vi "Unregister Subsystem.vi"(8 "error in (no error)":errorcluster, 9 "RegistryKey":string, 10 "JKI SMO":refnum<class "SMO.lvclass">) -> (0 "error out":errorcluster, 2 "JKI SMO out":refnum<class "SMO.lvclass">)   [LabVIEW 2021, in "smo.lvlib" / "Registry-SMO.lvclass"]
uses:
  Registry-SMO.lvclass
  SMO/SMO.lvclass
  SMO/SMO.lvclass/SMO.ctl
  Support/Attribute.Identity/Attribute.Identity.lvclass/Attribute.Identity.ctl
  Registry-SMO.lvclass/Registry-SMO.ctl
  SMO/Private/GetVariant(Attr).vi
  Support/Attribute.Identity/Read UniqueName.vi
  Support/Attribute.Identity/Read Given Name.vi
  Support/Attribute.Identity/Read ProspectiveOwner.vi
  SMO/Private/ReftoDVR--SMO.vi
  Support/Attribute.Identity/Attribute.Identity.lvclass
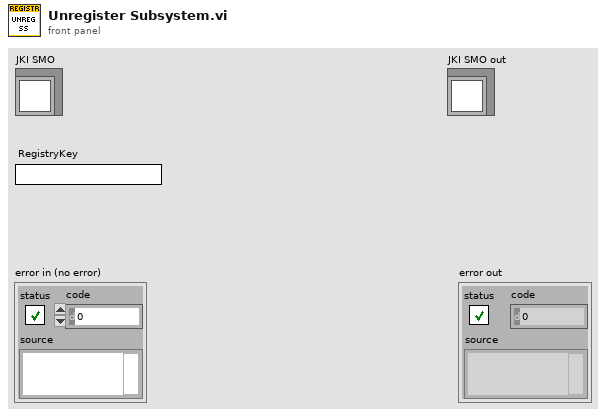
[diagram p1: front panel]
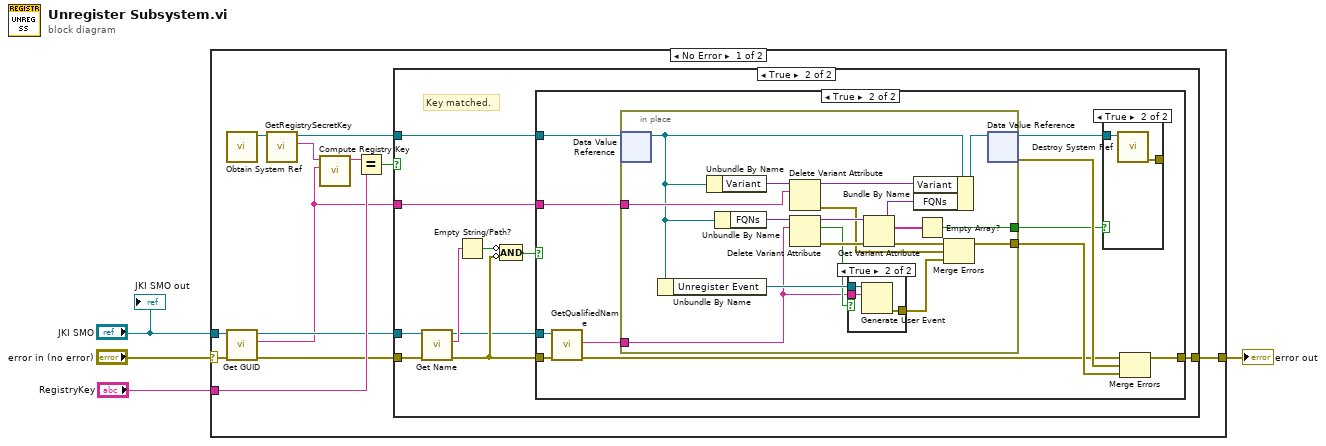
[diagram p0: block diagram]
diagram:
  n1 = case shown="No Error" "error in (no error)" {
    selector: "error in (no error)" -> [w15 w63]
    tunnel: [w16 w63] -> w3
    tunnel: "JKI SMO" -> [w14 _]
    tunnel: "RegistryKey" -> [w13 _]
    frame No Error {
      n2 = call "Obtain System Ref.vi"() -> ("JKI SMO System"=w10:refnum<data-value>)  [unwired: 10 in, 1 out]
      n3 = call "Get GUID.vi"("error in (no error)"=w15, "SMO"=w14) -> ("error out"=w12:errorcluster, "GUID"=w5:string, "SMO out"=w11:refnum<class "SMO.lvclass">)  [unwired: 7 in]
      n4 = call "GetRegistrySecretKey.vi"("Registry-SMO in"=w10) -> ("SecretKey"=w8:string, "Registry-SMO out"=w9:refnum<data-value>)  [unwired: 9 in]
      n5 = call "Compute Registry Key.vi"("SMO GUID"=w5, "Registry's SecretKey"=w8) -> ("Registry Key"=w7:string)  [unwired: 9 in]
      n6 = Equal?(x=w7, y=w13) -> (x = y?=w6:bool)
      n7 = case shown="True" w6 {
        tunnel: [w17 w27] -> w16
        tunnel: w12 -> [w17 w22]
        tunnel: w11 -> [_ w21]
        tunnel: w9 -> [_ w20]
        tunnel: w5 -> [_ w19]
        frame False {
          # "Registry Key does not match. Cannot unregister SMO"
        }
        frame True {
          # "Key matched."
          n8 = call "Get Name.vi"("error in (no error)"=w22, "SMO"=w21) -> ("error out"=w23:errorcluster, "Name"=w26:string, "SMO out"=w18:refnum<class "SMO.lvclass">)  [unwired: 5 in, 2 out]
          n9 = Empty String/Path?(string/path=w26) -> (empty?=w25:bool)
          n10 = Compound Arithmetic op=AND(invert w25, invert w23) -> (w24:bool)
          n11 = case shown="True" w24 {
            tunnel: [w28 w37] -> w27
            tunnel: w23 -> [w28 w32]
            tunnel: w20 -> [_ w36]
            tunnel: w19 -> [_ w33]
            tunnel: w18 -> [_ w30]
            frame False {
            }
            frame True {
              n12 = call "GetQualifiedName.vi"("error in (no error)"=w32, "SMO"=w30) -> ("error out"=w31:errorcluster, "Qualified Name"=w29:string)  [unwired: 7 in, 1 out]
              n13 = in-place {
                in-place-border: [w48] -> w38
                in-place-border: [w58] -> w34
                in-place-border: w33 -> [w55]
                in-place-border: w29 -> [w44]
                n14 = in-place-dvr #1(w36) -> (w43:refnum<class "Registry-SMO.lvclass">)  [unwired: 1 out]
                n15 = Unbundle By Name(w43) -> ("Unregister Event"=w47:refnum<user-event>)
                n16 = Unbundle By Name(w43) -> ("Variant"=w57:variant)
                n17 = Unbundle By Name(w43) -> ("FQNs"=w54:variant)
                n18 = Delete Variant Attribute(6:w55, 7:w57) -> (0:w50:errorcluster, 3:w56:variant)  [unwired: 1 in, 1 out]
                n19 = Delete Variant Attribute(6:w44, 7:w54) -> (0:w52:errorcluster, 2:w46:bool, 3:w53:variant)  [unwired: 1 in]
                n20 = case shown="True" w46 {
                  tunnel: [_ w62] -> w45
                  tunnel: w47 -> [_ w61]
                  tunnel: w44 -> [_ w60]
                  frame False {
                  }
                  frame True {
                    n21 = Generate User Event(user event=w61, event data cluster=w60) -> (error out=w62:errorcluster)  [unwired: 2 in, 1 out]
                  }
                }
                n22 = Get Variant Attribute(Variant=w53, error in=w52) -> (duplicate Variant=w42:variant, names=w59:string[], error out=w49:errorcluster)  [unwired: 2 in, 1 out]
                n23 = Bundle By Name(cluster=w43, "Variant"=w56, "FQNs"=w42) -> (w51:refnum<class "Registry-SMO.lvclass">)
                n24 = Empty Array?(array=w59) -> (empty?=w58:bool)
                n25 = Merge Errors(w49, w50, w45) -> (w48:errorcluster)
                n26 = in-place-dvr #1(w51) -> (w35:refnum<data-value>, w39:errorcluster)
              }
              n27 = case shown="True" w34 {
                tunnel: w35 -> [_ w41]
                tunnel: [_ w40] -> _
                frame False {
                }
                frame True {
                  n28 = call "Destroy System Ref.vi"("JKI SMO System"=w41) -> ("error out"=w40:errorcluster)  [unwired: 10 in]
                }
              }
              n29 = Merge Errors(w31, w39, w38) -> (w37:errorcluster)
            }
          }
        }
      }
    }
    frame Error {
    }
  }
  "error out" <- w3
  "JKI SMO out" <- "JKI SMO"
